vi "relay message.vi"(10 "User Events":refnum<user-event>, 11 "queue ref":refnum<queue>) -> ()   [LabVIEW 2023, in "Publisher Subscriber.lvlib"]
uses:
  <userlib>/_Publisher Subscriber/Publisher Subscriber.lvlib
  <userlib>/_Publisher Subscriber/Controls/data cluster.ctl
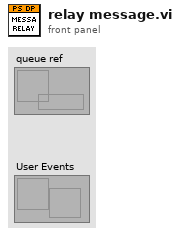
[diagram p1: front panel]
types:
  T1 = typedef "Publisher Subscriber.lvlib/data cluster.ctl" = cluster{"Command":string, "Data":variant}
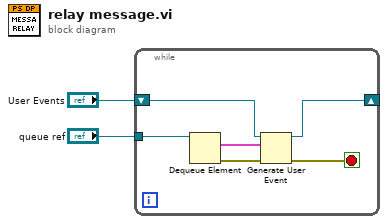
[diagram p0: block diagram]
diagram:
  n1 = while {
    shift-right: [w8] -> _
    shift-left: "User Events" -> [w6]
    tunnel: "queue ref" -> [w4]
    stop <- w7 stop-if-true
    n2 = Dequeue Element(queue=w4) -> (element=w3:T1, error out=w5:errorcluster)  [unwired: 2 in, 2 out]
    n3 = Generate User Event(user event=w6, event data cluster=w3, error in=w5) -> (user event out=w8:refnum<user-event>, error out=w7:errorcluster)  [unwired: 1 in]
  }
